vi "ErrorHandling.Extend.vi"(8 "error in":errorcluster, 10 "extra message part":string) -> (0 "error out":errorcluster)   [LabVIEW 2013]
doc: "Adds a piece of information to an error or warning. This is usually context information.\nThe text will not be added if no error or warning is in the wire.\n\nAn example could be the following situation. You have a subVI that converts strings to integers. This may fail, in which case it reports this:\n Could not interpret string as I32.\n String value: \"abc\"\nBut this does not indicate where it went wrong. So you can add this context information with this VI, creating:\n Could not interpret string as I32.\n String value: \"abc\"\n File: c:\\temp\\numerics.txt\n Line: 15"
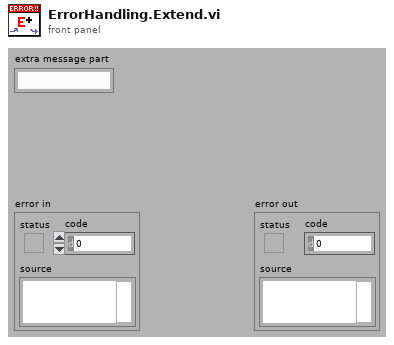
[diagram p1: front panel]
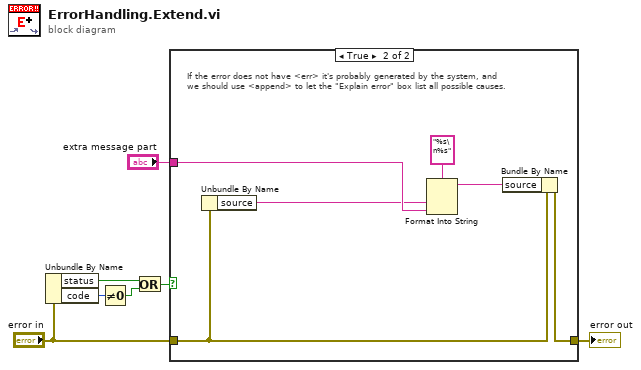
[diagram p0: block diagram]
diagram:
  n1 = Unbundle By Name("error in") -> ("status"=w6:bool, "code"=w4:i32)
  n2 = Not Equal To 0?(x=w4) -> (x != 0?=w3:bool)
  n3 = Or(x=w6, y=w3) -> (x .or. y?=w5:bool)
  n4 = case shown="True" w5 {
    tunnel: [w8 w14] -> w1
    tunnel: "error in" -> [w8 w13]
    tunnel: "extra message part" -> [_ w12]
    frame False {
    }
    frame True {
      # "If the error does not have <err> it's probably generated by the system, and\nwe should use <append> to let the \"Explain error\" box list all possible causes."
      n5 = Unbundle By Name(w13) -> ("source"=w10:string)
      n6 = Format Into String(format string="%s\n%s" ("string"), w10, w12) -> (resulting string=w11:string)  [unwired: 2 in, 1 out]
      n7 = Bundle By Name(cluster=w13, "source"=w11) -> (w14:errorcluster)
    }
  }
  "error out" <- w1
